vi "8-1.vi"() -> ()   [LabVIEW 2019, in "8.lvlib"]
uses:
  8.lvlib
panel:
  out "Number of 1,4,7,8":i32
  out "codes":string[][](array[string])
  out "patterns":string[][](array[string])
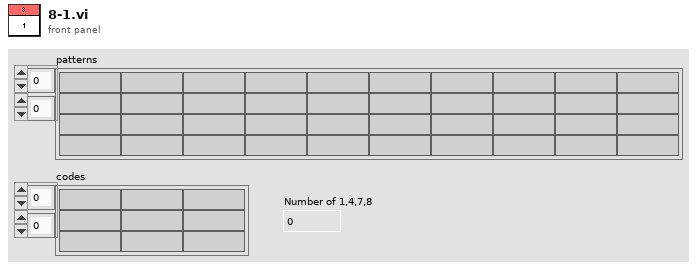
[diagram p1: front panel]
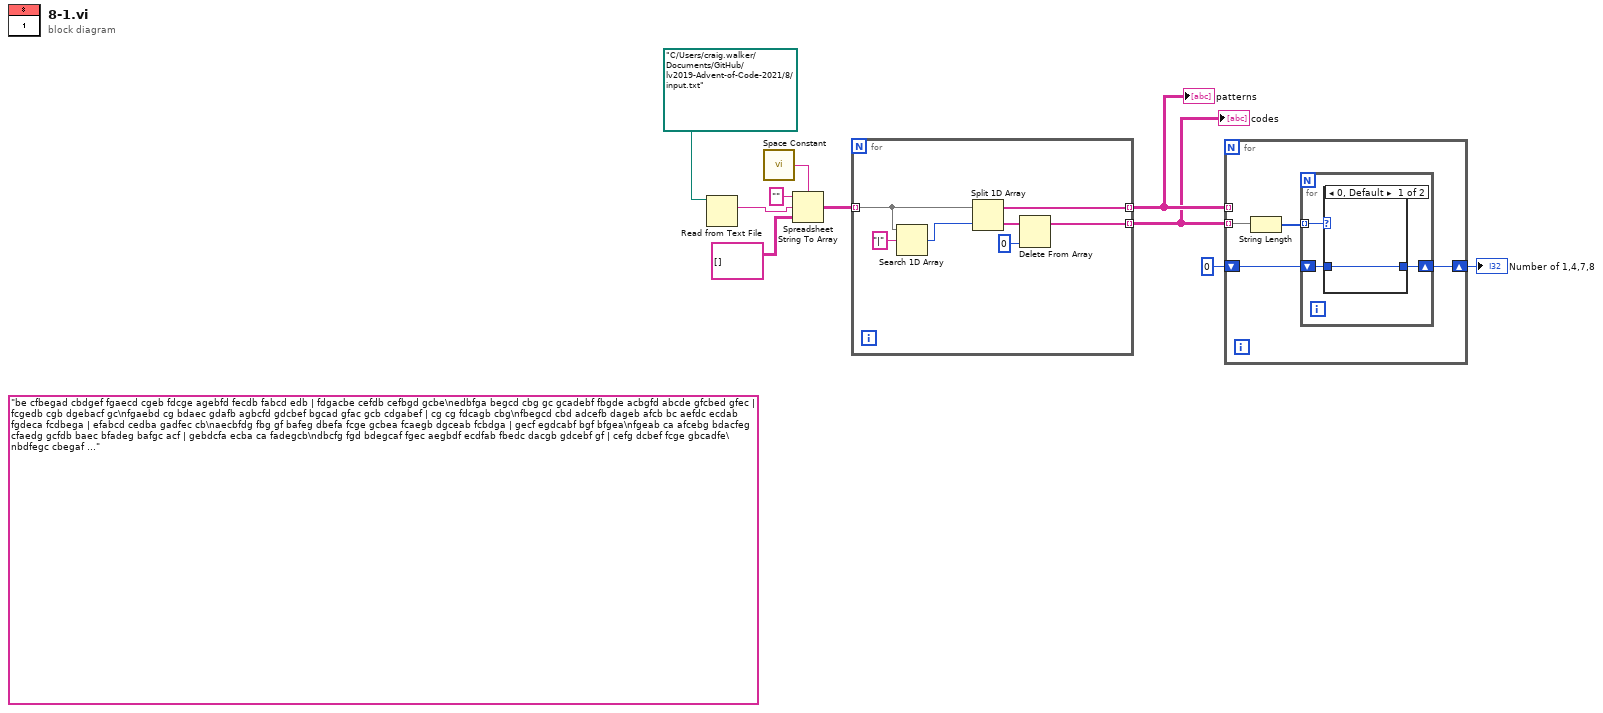
[diagram p0: block diagram]
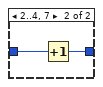
[diagram p2: hidden frame]
diagram:
  (unwired) "be cfbegad cbdgef fgaecd cgeb fdcge agebfd fecdb fabcd edb | fdgacbe cefdb cefbgd gcbe\nedbfga begcd cbg gc gcadebf fbgde acbgfd abcde gfcbed gfec | fcgedb cgb dgebacf gc\nfgaebd cg bdaec gdafb agbcfd gdcbef bgcad gfac gcb cdgabef | cg cg fdcagb cbg\nfbegcd cbd adcefb dageb afcb bc aefdc ecdab fgdeca fcdbega | efabcd cedba gadfec cb\naecbfdg fbg gf bafeg dbefa fcge gcbea fcaegb dgceab fcbdga | gecf egdcabf bgf bfgea\nfgeab ca afcebg bdacfeg cfaedg gcfdb baec bfadeg bafgc acf | gebdcfa ecba ca fadegcb\ndbcfg fgd bdegcaf fgec aegbdf ecdfab fbedc dacgb gdcebf gf | cefg dcbef fcge gbcadfe\nbdfegc cbegaf gecbf dfcage bdacg ed bedf ced adcbefg gebcd | ed bcgafe cdgba cbgef\negadfb cdbfeg cegd fecab cgb gbdefca cg fgcdab egfdb bfceg | gbdfcae bgc cg cgb\ngcafb gcf dcaebfg ecagb gf abcdeg gaef cafbge fdbac fegbdc | fgae cfgab fg bagce" ("element")
  n1 = Read from Text File(file (use dialog)=path "C:/Users/craig.walker/Documents/GitHub/lv2019-Advent-of-Code-2021/8/input.txt") -> (text=w1:string)  [unwired: 3 in, 3 out]
  n2 = call <vilib>:"Space Constant.vi"() -> ("String"=w8:string)
  n3 = Spreadsheet String To Array(delimiter (Tab)=w8, format string="", spreadsheet string=w1, array type (2D Dbl)=string[][] []) -> (array=w9:string[][])
  n4 = for {
    tunnel: w9 -> [w13] mode=indexing
    tunnel: [w12] -> w4 mode=indexing
    tunnel: [w11] -> w5 mode=indexing
    n5 = Search 1D Array(1D array=w13, element="|") -> (index of element=w16:i32)  [unwired: 1 in]
    n6 = Split 1D Array(array=w13, index=w16) -> (first subarray=w11:string[], second subarray=w15:string[])
    n7 = Delete From Array(array=w15, index=0) -> (array with subset deleted=w12:string[])  [unwired: 1 in, 1 out]
  }
  "patterns" <- w5
  "codes" <- w4
  n8 = for {
    tunnel: w5 -> [_] mode=indexing
    tunnel: w4 -> [w21] mode=indexing
    shift-right: [w18] -> w2
    shift-left: 0 -> [w19]
    n9 = String Length(string=w21) -> (length=w20:i32[])
    n10 = for {
      tunnel: w20 -> [w24] mode=indexing
      shift-right: [w22] -> w18
      shift-left: w19 -> [w23]
      n11 = case shown="0, Default" w24 {
        tunnel: w23 -> [w25 w27]
        tunnel: [w25 w26] -> w22
        frame 0, Default {
        }
        frame 2..4, 7 {
          n12 = Increment(x=w27) -> (x+1=w26:i32)
        }
      }
    }
  }
  "Number of 1,4,7,8" <- w2
